vi "Configure.vi"(8 "error in (no error)":errorcluster, 11 "AOTF in":refnum<class "AOTF.lvclass">) -> (0 "error out":errorcluster, 2 "cancelled?":bool, 3 "AOTF out":refnum<class "AOTF.lvclass">)   [LabVIEW 2012, in "AOTF.lvclass"]
doc: "The configure method configures the details for the RabbitMQ connection. \n\nIn the derived class, make a call to the parent for setting these parameters."
uses:
  AOTF.lvclass
  <vilib>/Utility/miscctls.llb/LVPointTypeDef.ctl
  AOTF.lvclass/AOTF.ctl
  <vilib>/Distrio/Murmex/Murmex/Murmex.lvclass
panel:
  in  "button::configure murmex":bool
  in  "button::ok":bool
  in  "button::cancel":bool
  in  "Tab Control":enum32{"AOTF", "Rotary stage"}(tab)
  in  "LUT638":path=path "D:/CLSM_Project/AOTF/561nm.txt" caption="LUT 561nm"
  in  "DO lines":tag
  in  "AO channel":tag
  in  "LUT561":path=path "D:/CLSM_Project/AOTF/561nm.txt" caption="LUT 561nm"
  in  "LUT515":path=path "D:/CLSM_Project/AOTF/515nm.txt" caption="LUT 515nm"
  in  "LUT491":path=path "D:/CLSM_Project/AOTF/491nm.txt" caption="LUT 491nm"
  in  "LUT445":path=path "D:/CLSM_Project/AOTF/445nm.txt" caption="LUT 445nm"
  in  "LUT405":path=path "D:/CLSM_Project/AOTF/405nm.txt" caption="LUT 405nm"
  in  "Controller S/N":i32
  in  "Florence angles":sgl[](array[numeric])
  in  "Prato angles":sgl[](array[numeric])
  # "RabbitMQ parameters"
  # "Window position"
  # "Florence"
  # "Prato"
  # "405 nm"
  # "445 nm"
  # "491 nm"
  # "515 nm"
  # "561 nm"
  # "638 nm"
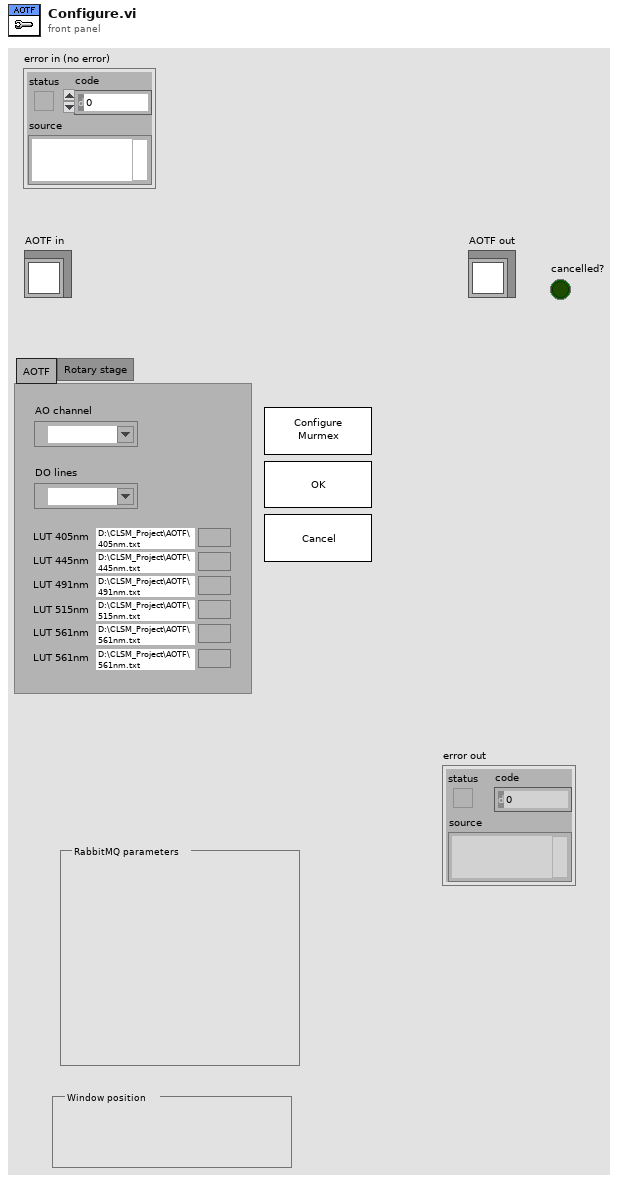
[diagram p1: front panel]
types:
  T1 = typedef "LVPointTypeDef.ctl" = cluster{"Horizontal":i16, "Vertical":i16}
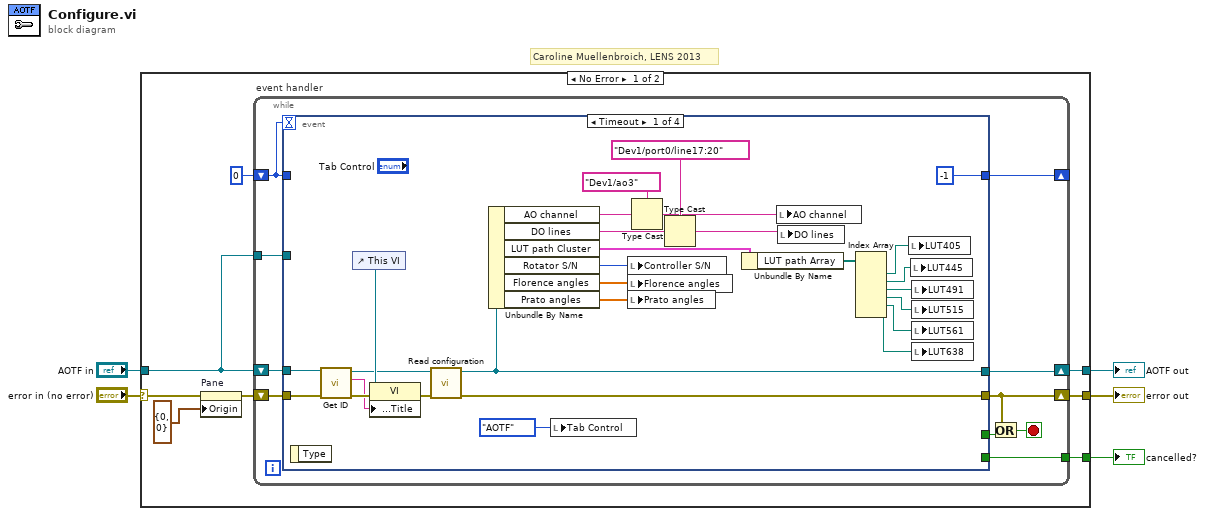
[diagram p0: block diagram]
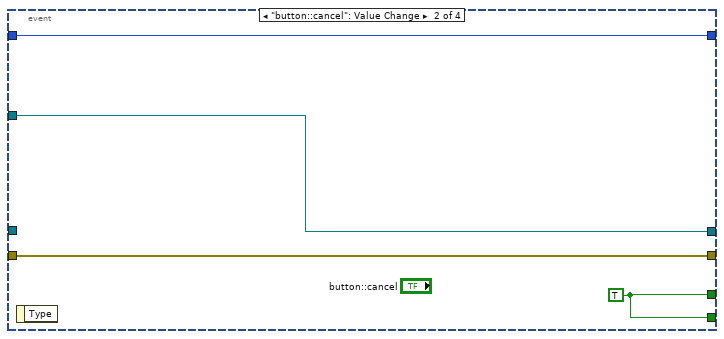
[diagram p2: hidden frame]
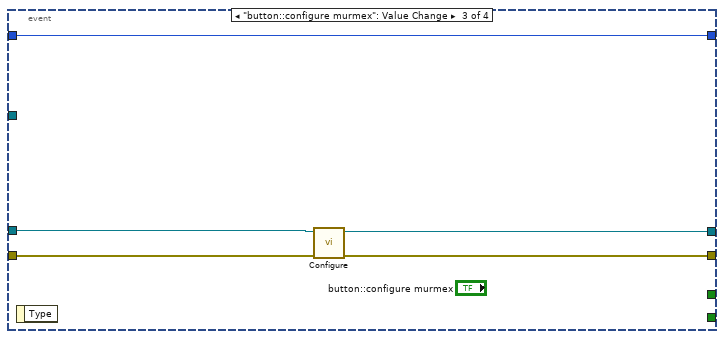
[diagram p3: hidden frame]
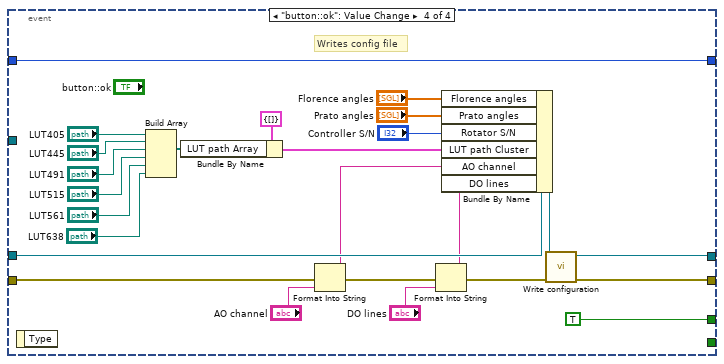
[diagram p4: hidden frame]
diagram:
  # "Caroline Muellenbroich, LENS 2013"
  n1 = case shown="No Error" "error in (no error)" {
    selector: "error in (no error)" -> [w11 w86]
    tunnel: "AOTF in" -> [w12 w87]
    tunnel: [w8 w86] -> w1
    tunnel: [w7 w87] -> w3
    tunnel: [w6 _] -> w2
    frame No Error {
      n2 = property on="Pane" class="Pane"(error in=w11, "Origin"=T1 {"Horizontal"=0, "Vertical"=0}) -> (error out=w10:errorcluster)  [unwired: 1 in, 1 out]
      n3 = while "event handler" {
        shift-right: [w23] -> _
        shift-left: 0 -> [w14]
        shift-right: [w19] -> w7
        shift-left: w12 -> [w22]
        tunnel: w12 -> [w21]
        shift-right: [w17] -> w8
        shift-left: w10 -> [w20]
        tunnel: [w15] -> w6
        stop <- w18 stop-if-true
        n4 = event shown="[0] Timeout" {
          selector: _ -> [_ _ _ _]
          dyn-events: _ -> [_ _ _ _]
          timeout: w14 -> [_ _ _ _]
          tunnel: w14 -> [_ w55 w60 w85]
          tunnel: [-1 w55 w60 w85] -> w23
          tunnel: w22 -> [w47 _ w57 w82]
          tunnel: w21 -> [_ w52 _ _]
          tunnel: w20 -> [w50 w53 w56 w76]
          tunnel: [w43 w52 w58 w83] -> w19
          tunnel: [w42 w53 w59 w84] -> w17
          tunnel: [_ w54 _ TRUE ("force loading?")] -> w16
          tunnel: [_ w54 _ _] -> w15
          event Timeout {
            n5 = event-data() -> ()  [unwired: 1 in, 1 out]
            n6 = call <vilib>:"Get ID.vi"("error in (no error)"=w50, "Murmex in"=w47) -> ("error out"=w48:errorcluster, "component id"=w46:string, "Murmex out"=w44:refnum<class "AOTF.lvclass">)  [unwired: 7 in]
            n7 = control-ref of="This VI"() -> (w49:refnum<vi>)
            n8 = property class="VI"(reference=w49, error in=w48, "Front Panel.Title"=w46) -> (error out=w45:errorcluster)  [unwired: 1 out]
            n9 = call <vilib>:"Read configuration.vi"("error in (no error)"=w45, "Murmex in"=w44) -> ("error out"=w42:errorcluster, "Murmex out"=w43:refnum<class "AOTF.lvclass">)  [unwired: 7 in, 1 out]
            n10 = Unbundle By Name(w43) -> ("AO channel"=w38:string, "DO lines"=w37:string, "LUT path Cluster"=w41:cluster{"LUT path Array":path[]}, "Rotator S/N"=w31:i32, "Florence angles"=w30:sgl[], "Prato angles"=w29:sgl[])
            n11 = local write "Tab Control"(enum32{"AOTF", "Rotary stage"}."AOTF" ("Tab Control")) -> ()
            n12 = local write "Controller S/N"(w31) -> ()
            n13 = local write "Florence angles"(w30) -> ()
            n14 = local write "Prato angles"(w29) -> ()
            n15 = Type Cast(type=tag "Dev1/ao3" ("AO channel"), x=w38) -> (*(type *) &x=w34:tag)
            n16 = Type Cast(type=tag "Dev1/port0/line17:20" ("DO lines"), x=w37) -> (*(type *) &x=w33:tag)
            n17 = Unbundle By Name(w41) -> ("LUT path Array"=w40:path[])
            n18 = local write "AO channel"(w34) -> ()
            n19 = local write "DO lines"(w33) -> ()
            n20 = Index Array(array=w40) -> (element #1=w39:path, element #2=w27:path, element #3=w26:path, element #4=w25:path, element #5=w24:path, element #6=w28:path)  [unwired: 6 in]
            n21 = local write "LUT405"(w39) -> ()
            n22 = local write "LUT445"(w27) -> ()
            n23 = local write "LUT491"(w26) -> ()
            n24 = local write "LUT515"(w25) -> ()
            n25 = local write "LUT561"(w24) -> ()
            n26 = local write "LUT638"(w28) -> ()
          }
          event "button::cancel": Value Change {
            w54 = TRUE ("force loading?")
            n27 = event-data() -> ()  [unwired: 1 in, 1 out]
          }
          event "button::configure murmex": Value Change {
            n28 = event-data() -> ()  [unwired: 1 in, 1 out]
            n29 = call-parent "Configure.vi"("error in (no error)"=w56, "Murmex in"=w57) -> ("error out"=w59:errorcluster, "Murmex out"=w58:refnum<class "AOTF.lvclass">)  [unwired: 7 in, 1 out]
          }
          event "button::ok": Value Change {
            # "Writes config file"
            n30 = event-data() -> ()  [unwired: 1 in, 1 out]
            n31 = Build Array("LUT405", "LUT445", "LUT491", "LUT515", "LUT561", "LUT638") -> (w79:path[])
            n32 = Bundle By Name(cluster=cluster{"LUT path Array":path[]} {"LUT path Array"=[]} ("Confiugration cluster.LUT path Cluster"), "LUT path Array"=w79) -> (w69:cluster{"LUT path Array":path[]})
            n33 = Format Into String(error in=w76, "AO channel") -> (resulting string=w71:string, error out=w75:errorcluster)  [unwired: 2 in]
            n34 = Format Into String(error in=w75, "DO lines") -> (resulting string=w72:string, error out=w74:errorcluster)  [unwired: 2 in]
            n35 = Bundle By Name(cluster=w82, "Florence angles"="Florence angles", "Prato angles"="Prato angles", "Rotator S/N"="Controller S/N", "LUT path Cluster"=w69, "AO channel"=w71, "DO lines"=w72) -> (w81:refnum<class "AOTF.lvclass">)
            n36 = call <vilib>:"Write configuration.vi"("error in (no error)"=w74, "Murmex in"=w81) -> ("error out"=w84:errorcluster, "Murmex out"=w83:refnum<class "AOTF.lvclass">)  [unwired: 8 in]
          }
        }
        n37 = Or(x=w17, y=w16) -> (x .or. y?=w18:bool)
      }
    }
    frame Error {
    }
  }
  "error out" <- w1
  "AOTF out" <- w3
  "cancelled?" <- w2
